vi "pylights.vi"() -> ()   [LabVIEW 2021]
panel:
  out "Cluster 2":cluster{"Red":bool, "Amber":bool, "Green":bool}
  out "Array 2":bool[][](array[boolean])
  in  "TFL":cluster{"red":bool, "amber":bool, "green":bool}
  in  "Array":bool[][](array[boolean])
  in  "Boolean 2":bool
  in  "Boolean":bool
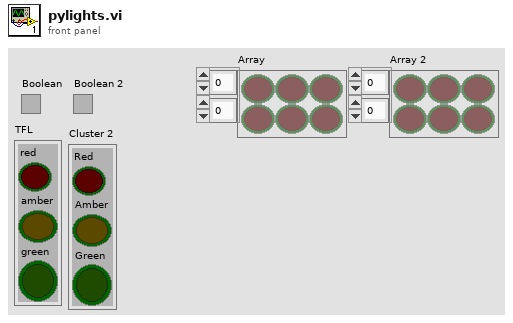
[diagram p1: front panel]
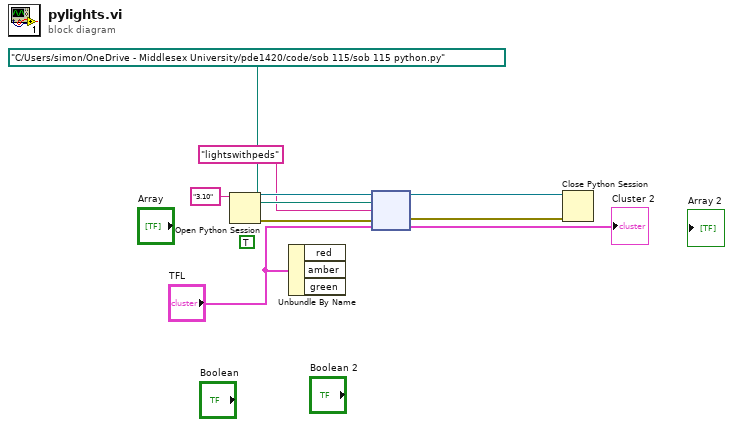
[diagram p0: block diagram]
diagram:
  (unwired) TRUE
  n1 = Open Python Session(python version="3.10" ("Python version")) -> (session out=w8:refnum<k35>, error out=w7:errorcluster)  [unwired: 2 in]
  n2 = Unbundle By Name("TFL") -> ()  [unwired: 3 out]
  n3 = node(w8, path "C:/Users/simon/OneDrive - Middlesex University/pde1420/code/sob 115/sob 115 python.py" ("module path"), "lightswithpeds" ("function name"), w7, "TFL") -> (w3:refnum<k35>, w6:errorcluster, →"Cluster 2":cluster{"red":bool, "amber":bool, "green":bool})  [unwired: 2 out]
  n4 = Close Python Session(session in=w3, error in=w6) -> ()  [unwired: 1 out]
